vi "Torque forearm and backarm.vi"() -> ()   [LabVIEW 2017]
panel:
  out "Torque of forearm":dbl format="%#_13g"
  in  "Boolean":bool=TRUE
  out "Torque of shoulder":dbl format="%#_13g"
  in  "Weight of cube":dbl format="%#_13g"
  in  "Length of four":dbl format="%#_13g"
  in  "Weight of three":dbl format="%#_13g"
  in  "Beta":dbl format="%#_13g"
  in  "Length of three":dbl format="%#_13g"
  out "Phi":dbl format="%#_13g"
  in  "Length of two":dbl format="%#_13g"
  in  "Weight of 1":dbl format="%#_13g"
  in  "Alpha":dbl format="%#_13g"
  in  "Length of one":dbl format="%#_13g"
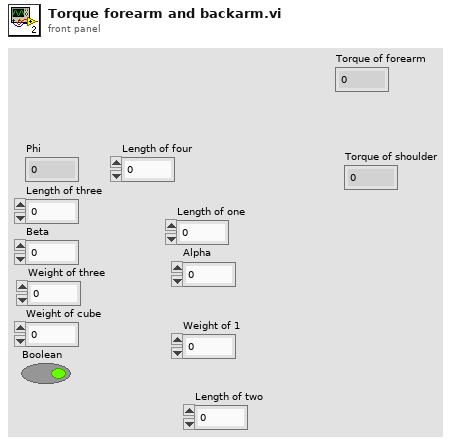
[diagram p1: front panel]
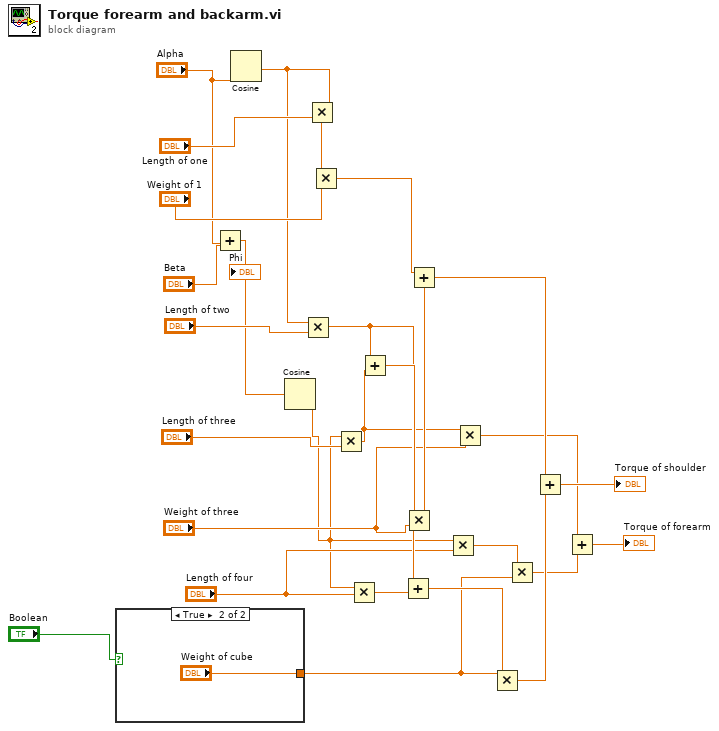
[diagram p0: block diagram]
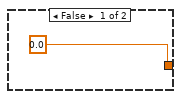
[diagram p2: hidden frame]
diagram:
  n1 = case shown="True" "Boolean" {
    tunnel: [0.0 "Weight of cube"] -> w5
    frame False {
    }
    frame True {
    }
  }
  n2 = Add(x="Alpha", y="Beta") -> (x+y=w20:dbl)
  "Phi" <- w20
  n3 = Cosine(x="Alpha") -> (cos(x)=w21:dbl)
  n4 = Cosine(x=w20) -> (cos(x)=w6:dbl)
  n5 = Multiply(x=w21, y="Length of two") -> (x*y=w15:dbl)
  n6 = Multiply(x=w21, y="Length of one") -> (x*y=w26:dbl)
  n7 = Multiply(x=w26, y="Weight of 1") -> (x*y=w19:dbl)
  n8 = Multiply(x=w6, y="Length of three") -> (x*y=w9:dbl)
  n9 = Multiply(x=w6, y="Length of four") -> (x*y=w16:dbl)
  n10 = Add(x=w15, y=w9) -> (x+y=w18:dbl)
  n11 = Add(x=w15, y=w16) -> (x+y=w14:dbl)
  n12 = Multiply(x=w18, y="Weight of three") -> (x*y=w17:dbl)
  n13 = Add(x=w19, y=w17) -> (x+y=w12:dbl)
  n14 = Multiply(x=w6, y="Length of four") -> (x*y=w4:dbl)
  n15 = Multiply(x=w9, y="Weight of three") -> (x*y=w3:dbl)
  n16 = Multiply(x=w14, y=w5) -> (x*y=w13:dbl)
  n17 = Multiply(x=w4, y=w5) -> (x*y=w2:dbl)
  n18 = Add(x=w12, y=w13) -> (x+y=→"Torque of shoulder":dbl)
  n19 = Add(x=w3, y=w2) -> (x+y=→"Torque of forearm":dbl)
